vi "Within Msg Set.vi"(9 "Msg":refnum<class "Msg.lvclass">, 10 "Msg Set":T1) -> (2 "Within Msg Set":bool)   [LabVIEW 2025, in "jettl.lvlib"]
uses:
  jettl.lvlib
  Msg Set.ctl
  Msg/Msg.lvclass
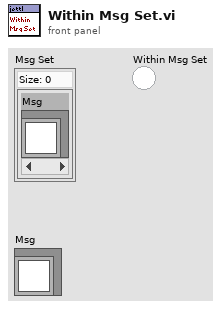
[diagram p1: front panel]
types:
  T1 = typedef "jettl.lvlib/Msg Set.ctl" = set{refnum<class "Msg.lvclass">}
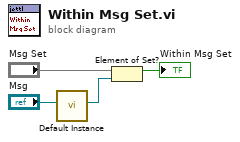
[diagram p0: block diagram]
diagram:
  n1 = call "Default Instance.vi"("Instance"="Msg") -> ("Default Instance"=w1:refnum<class "Msg.lvclass">)  [unwired: 10 in]
  n2 = Element of Set?(10:w1, 11:"Msg Set") -> (3:→"Within Msg Set":bool)
